vi "BNC555.Read Sys To Parameters.vi"(0 "i ref in":refnum<vi>, 2 "Parameter":T1(ring), 3 "Sys State":bool, 5 "error in (no error)":errorcluster) -> (14 "i ref out":refnum<vi>, 19 "error out":errorcluster)   [LabVIEW 2014, in "BNC555.lvlib"]
doc: "This VI queries the device state. The result is indicated as the GUI element and published as a dim service status (3: failure in case of an error, 1: off resp. 2: on).\n\nDue to a firmware bug, the To state is not read out. Therefore the input \"Sys State\" has to be used; here the hardware is not asked but set to the required value which is published as DIM service as written above and stored to ownb attributes."
uses:
  BNC555.lvlib
  CSPhelix/PH_StatusHandler/PH_StatusHandler.Status.ctl
  CSPhelix/PH_StatusHandler/PH_StatusHandler.lvlib
  non_GPL/instr.lib/BNC555/BNC555 - Driver np.lvlib
  lib.lib/DimLVEvent/LVDimInterface/LVDimInterface.lvlib
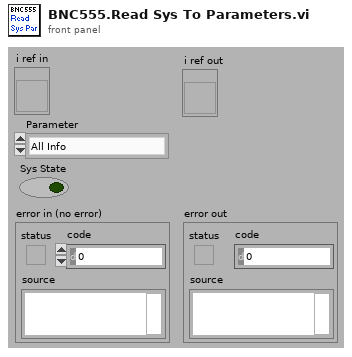
[diagram p1: front panel]
types:
  T1 = enum16{"All Info", "State", "Period", "Oscillator", "Mode", "Trigger"}
  T2 = typedef "BNC555.lvlib/BNC555.i attribute.ctl" = cluster{"Information":cluster{"VISA resource name":refnum<visa-resource-name>, "Baud Rate (1:9600)":u16}, "Channel Array":T3[], "System":T4, "GUI Refs":cluster{"Delete":refnum<vi>, "Information":refnum<vi>, "System":refnum<vi>, "Channel Array":refnum<vi>, "Device Error":refnum<vi>, "Instr Driver Revision":refnum<vi>, "Instr Firmware Revision":refnum<vi>, "Instr Option":refnum<vi>, "Self-Test Response":refnum<vi>}, "Service IDs Channelinfo":i32[], "Service ID T0 Mode":i32}
  T3 = typedef "BNC555 - Driver np.lvlib/BNC555 All Chan Parameters.ctl" = cluster{"Chan #":i32, "Chan State":bool, "Chan Delay":dbl, "Chan Width":dbl, "Chan Mode":enum16{"Normal", "Single", "Burst", "Divide by N"}, "Chan Burst #":u32, "Chan Divide #":u32, "Chan Pol Out":enum16{"Normal", "Complement", "Inverted"}, "Chan Level Out":enum16{"TTL", "Adjustable", "35 Volt"}, "Chan Lev Adjust":dbl, "Chan Gate Pol":enum16{"Normal", "Complement", "Inverted"}, "Chan Gate State":bool}
  T4 = typedef "BNC555 - Driver np.lvlib/BNC555 All Sys Parameters.ctl" = cluster{"Sys Period":dbl, "Sys Oscillator":bool, "Sys Mode":enum16{"Normal", "Single", "Burst", "Duty Cycle"}, "Sys Burst #":u32, "Sys DC On":u32, "Sys DC Off":u32, "Sys Trig Mode":enum16{"Disabled", "Triggered", "Gated"}, "Sys Trig Lev":dbl, "Sys Gate State":bool, "Sys Trig Edge":bool, "Sys State":bool}
  T5 = enum16{"All Info", "State", "Period", "Oscillator", "Mode", "Trigger"}[]
  T6 = typedef "PH_StatusHandler.lvlib/PH_StatusHandler.Status.ctl" = i16
  T7 = enum16{"Normal", "Single", "Burst", "Duty Cycle"}
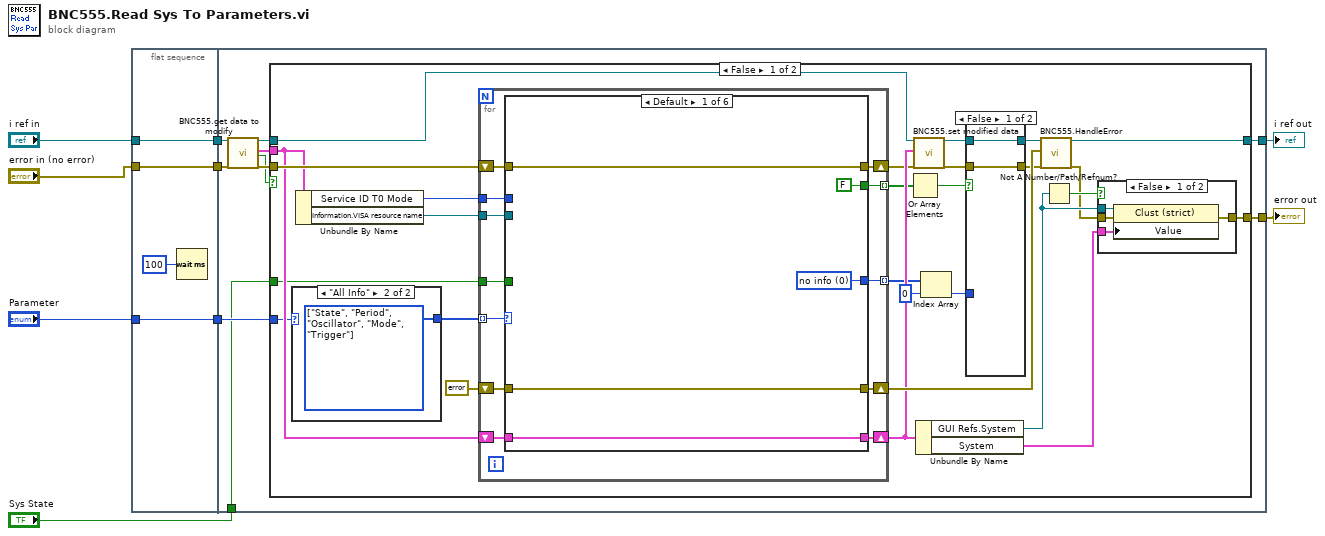
[diagram p0: block diagram]
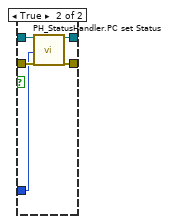
[diagram p2: hidden frame]
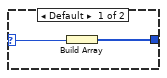
[diagram p3: hidden frame]
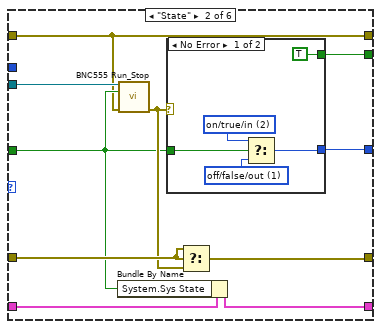
[diagram p4: hidden frame]
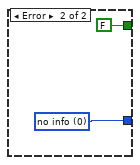
[diagram p5: hidden frame]
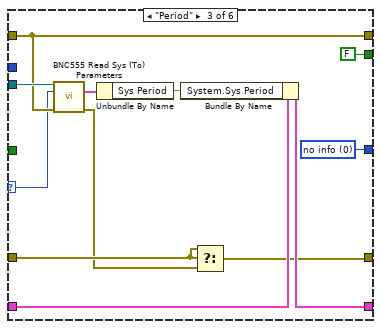
[diagram p6: hidden frame]
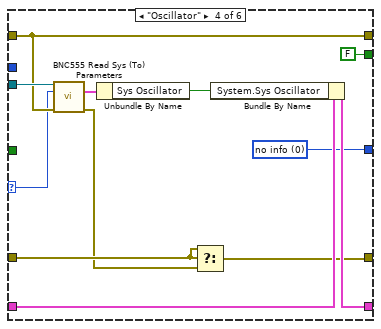
[diagram p7: hidden frame]
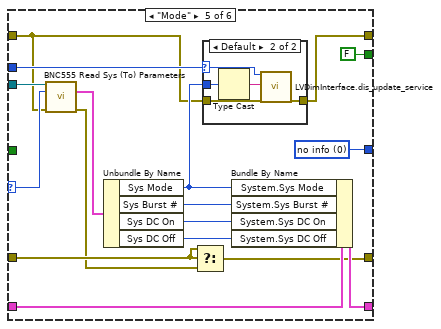
[diagram p8: hidden frame]
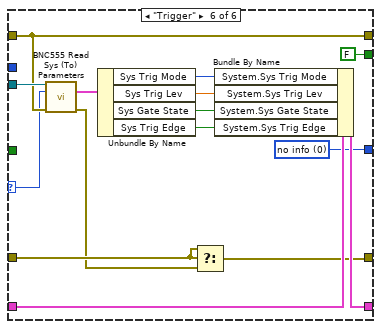
[diagram p10: hidden frame]
diagram:
  n1 = flat-sequence {
    tunnel: "Parameter" -> [w11]
    tunnel: "error in (no error)" -> [w12]
    tunnel: "i ref in" -> [w13]
    tunnel: [w13] -> w4
    tunnel: [w12] -> w3
    tunnel: [w11] -> w2
    tunnel: [w18] -> w7
    tunnel: [w17] -> w6
    tunnel: w4 -> [w23]
    tunnel: w3 -> [w22]
    tunnel: w2 -> [w15]
    tunnel: "Sys State" -> [w14]
    frame #0 {
      n2 = Wait (ms)(milliseconds to wait=u32 100) -> ()  [unwired: 1 out]
    }
    frame #1 {
      n3 = call "BNC555.get data to modify.vi"("i ref in"=w23, "error in (no error)"=w22) -> ("i ref out"=w19:refnum<vi>, "i attribute"=w21:T2, "timed out"=w16:bool, "error out"=w20:errorcluster)  [unwired: 14 in]
      n4 = case shown="False" w16 {
        tunnel: w21 -> [w43 _]
        tunnel: w20 -> [w50 w162]
        tunnel: w19 -> [w24 w163]
        tunnel: [w35 w163] -> w18
        tunnel: [w46 w162] -> w17
        tunnel: w15 -> [w41 _]
        tunnel: w14 -> [w40 _]
        frame False {
          n5 = case shown="\"All Info\"" w41 {
            selector: w41 -> [w59 _]
            tunnel: [w58 w60] -> w44
            frame Default {
              n6 = Build Array(w59) -> (w58:T5)
            }
            frame "All Info" {
              w60 = T5 [enum."State", enum."Period", enum."Oscillator", enum."Mode", enum."Trigger"] items=["All Info", "State", "Period", "Oscillator", "Mode", "Trigger"]
            }
          }
          n7 = Unbundle By Name(w43) -> ("Service ID T0 Mode"=w39:i32, "Information.VISA resource name"=w49:refnum<visa-resource-name>)
          n8 = for {
            tunnel: w49 -> [w71]
            shift-right: [w69] -> w36
            shift-left: w50 -> [w72]
            tunnel: w44 -> [w68] mode=indexing
            shift-right: [w67] -> w38
            shift-left: w43 -> [w66]
            shift-right: [w70] -> w47
            shift-left: errorcluster {"status"=FALSE, "code"=0, "source"=""} ("error out") -> [w65]
            tunnel: w40 -> [w64]
            tunnel: w39 -> [w63]
            tunnel: [w62] -> w29 mode=indexing
            tunnel: [w61] -> w26 mode=indexing
            n9 = case shown="Default" w68 {
              selector: w68 -> [_ _ w97 w109 w128 w147]
              tunnel: w72 -> [w76 w78 w104 w116 w119 w154]
              tunnel: w71 -> [_ w87 w106 w118 w135 w156]
              tunnel: [w75 w82 w100 w112 w131 w150] -> w70
              tunnel: [w76 w78 w104 w116 w124 w154] -> w69
              tunnel: [w77 w86 w101 w113 w132 w151] -> w67
              tunnel: w66 -> [w77 w85 w102 w114 w133 w152]
              tunnel: w65 -> [w75 w84 w99 w111 w130 w149]
              tunnel: w64 -> [_ w81 _ _ _ _]
              tunnel: w63 -> [_ _ _ _ w122 _]
              tunnel: [w74 w80 w96 w108 w121 w143] -> w62
              tunnel: [FALSE w79 FALSE FALSE FALSE FALSE] -> w61
              frame Default {
                w74 = T6 0 items=["no info", "off/false/out", "on/true/in", "Failure", "Alarm", "Status 1", "Status 2", "Status 3"] ("Status")
              }
              frame "State" {
                n10 = Bundle By Name(cluster=w85, "System.Sys State"=w81) -> (w86:T2)
                n11 = call "BNC555 Run_Stop.vi"("VISA resource"=w87, "Start\\Stop (T:Run)"=w81, "error in (no error)"=w78) -> ("error out"=w83:errorcluster)  [unwired: 11 in, 1 out]
                n12 = case shown="No Error" w83 {
                  tunnel: w81 -> [w92 _]
                  tunnel: [w89 w94] -> w80
                  tunnel: [TRUE FALSE] -> w79
                  frame No Error {
                    w91 = T6 1 items=["no info", "off/false/out", "on/true/in", "Failure", "Alarm", "Status 1", "Status 2", "Status 3"] ("Status")
                    w90 = T6 2 items=["no info", "off/false/out", "on/true/in", "Failure", "Alarm", "Status 1", "Status 2", "Status 3"] ("Status")
                    n13 = Select(t=w90, s=w92, f=w91) -> (s? t:f=w89:T6)
                  }
                  frame Error {
                    w94 = T6 0 items=["no info", "off/false/out", "on/true/in", "Failure", "Alarm", "Status 1", "Status 2", "Status 3"] ("Status")
                  }
                }
                n14 = Select(t=w84, s=w84, f=w83) -> (s? t:f=w82:errorcluster)
              }
              frame "Period" {
                w96 = T6 0 items=["no info", "off/false/out", "on/true/in", "Failure", "Alarm", "Status 1", "Status 2", "Status 3"] ("Status")
                n15 = call "BNC555 Read Sys (To) Parameters.vi"("VISA resource"=w106, "Parameter (1:State)"=w97, "error in (no error)"=w104) -> ("System Paramaters"=w105:T4, "error out"=w98:errorcluster)  [unwired: 10 in, 1 out]
                n16 = Unbundle By Name(w105) -> ("Sys Period"=w103:dbl)
                n17 = Bundle By Name(cluster=w102, "System.Sys Period"=w103) -> (w101:T2)
                n18 = Select(t=w99, s=w99, f=w98) -> (s? t:f=w100:errorcluster)
              }
              frame "Oscillator" {
                w108 = T6 0 items=["no info", "off/false/out", "on/true/in", "Failure", "Alarm", "Status 1", "Status 2", "Status 3"] ("Status")
                n19 = call "BNC555 Read Sys (To) Parameters.vi"("VISA resource"=w118, "Parameter (1:State)"=w109, "error in (no error)"=w116) -> ("System Paramaters"=w117:T4, "error out"=w110:errorcluster)  [unwired: 10 in, 1 out]
                n20 = Unbundle By Name(w117) -> ("Sys Oscillator"=w115:bool)
                n21 = Select(t=w111, s=w111, f=w110) -> (s? t:f=w112:errorcluster)
                n22 = Bundle By Name(cluster=w114, "System.Sys Oscillator"=w115) -> (w113:T2)
              }
              frame "Mode" {
                w121 = T6 0 items=["no info", "off/false/out", "on/true/in", "Failure", "Alarm", "Status 1", "Status 2", "Status 3"] ("Status")
                n23 = call "BNC555 Read Sys (To) Parameters.vi"("VISA resource"=w135, "Parameter (1:State)"=w128, "error in (no error)"=w119) -> ("System Paramaters"=w134:T4, "error out"=w129:errorcluster)  [unwired: 10 in, 1 out]
                n24 = Unbundle By Name(w134) -> ("Sys Mode"=w123:T7, "Sys Burst #"=w127:u32, "Sys DC On"=w126:u32, "Sys DC Off"=w125:u32)
                n25 = Select(t=w130, s=w130, f=w129) -> (s? t:f=w131:errorcluster)
                n26 = case shown="Default" w122 {
                  selector: w122 -> [_ w137]
                  tunnel: w119 -> [w136 w140]
                  tunnel: [w136 w139] -> w124
                  tunnel: w123 -> [_ w138]
                  frame -1 {
                  }
                  frame Default {
                    n27 = Type Cast(x=w138) -> (*(type *) &x=w141:string)  [unwired: 1 in]
                    n28 = call "LVDimInterface.dis_update_service.vi"("my_serviceID"=w137, "data"=w141, "error in (no error)"=w140) -> ("error out"=w139:errorcluster)  [unwired: 14 in, 2 out]
                  }
                }
                n29 = Bundle By Name(cluster=w133, "System.Sys Mode"=w123, "System.Sys Burst #"=w127, "System.Sys DC On"=w126, "System.Sys DC Off"=w125) -> (w132:T2)
              }
              frame "Trigger" {
                w143 = T6 0 items=["no info", "off/false/out", "on/true/in", "Failure", "Alarm", "Status 1", "Status 2", "Status 3"] ("Status")
                n30 = call "BNC555 Read Sys (To) Parameters.vi"("VISA resource"=w156, "Parameter (1:State)"=w147, "error in (no error)"=w154) -> ("System Paramaters"=w155:T4, "error out"=w148:errorcluster)  [unwired: 10 in, 1 out]
                n31 = Unbundle By Name(w155) -> ("Sys Trig Mode"=w153:enum16{"Disabled", "Triggered", "Gated"}, "Sys Trig Lev"=w146:dbl, "Sys Gate State"=w145:bool, "Sys Trig Edge"=w144:bool)
                n32 = Select(t=w149, s=w149, f=w148) -> (s? t:f=w150:errorcluster)
                n33 = Bundle By Name(cluster=w152, "System.Sys Trig Mode"=w153, "System.Sys Trig Lev"=w146, "System.Sys Gate State"=w145, "System.Sys Trig Edge"=w144) -> (w151:T2)
              }
            }
          }
          n34 = Or Array Elements(Boolean array=w26) -> (logical OR=w25:bool)
          n35 = call "BNC555.set modified data.vi"("i ref in"=w24, "i attribute"=w38, "error in (no error)"=w36) -> ("i ref out"=w33:refnum<vi>, "error out"=w31:errorcluster)  [unwired: 15 in]
          n36 = Unbundle By Name(w38) -> ("GUI Refs.System"=w37:refnum<vi>, "System"=w45:T4)
          n37 = Index Array(array=w29, index=0) -> (element=w27:T6)
          n38 = case shown="False" w25 {
            tunnel: w33 -> [w52 w57]
            tunnel: [w52 w56] -> w32
            tunnel: w31 -> [w51 w55]
            tunnel: [w51 w54] -> w30
            tunnel: w27 -> [_ w53]
            frame False {
            }
            frame True {
              n39 = call "PH_StatusHandler.PC set Status.vi"("i ref in"=w57, "Status"=w53, "error in (no error)"=w55) -> ("i ref out"=w56:refnum<vi>, "error out"=w54:errorcluster)  [unwired: 15 in]
            }
          }
          n40 = call "BNC555.HandleError.vi"("i ref in"=w32, "Device error"=w47, "error in (no error)"=w30) -> ("i ref out"=w35:refnum<vi>, "error out"=w34:errorcluster)  [unwired: 15 in]
          n41 = Not A Number/Path/Refnum?(number/path/refnum=w37) -> (NaN/Path/Refnum?=w48:bool)
          n42 = case shown="False" w48 {
            tunnel: [w160 w161] -> w46
            tunnel: w45 -> [w159 _]
            tunnel: w34 -> [w158 w161]
            tunnel: w37 -> [w157 _]
            frame False {
              n43 = property class="Clust (strict)"(reference=w157, error in=w158, "Value"=w159) -> (error out=w160:errorcluster)  [unwired: 1 out]
            }
            frame True {
            }
          }
        }
        frame True {
        }
      }
    }
  }
  "i ref out" <- w7
  "error out" <- w6
